vi "connect.vi"(0 "username":string="user", 5 "password":string="password", 7 "host":string="localhost", 9 "port":i32=33060, 11 "error in (no error)":errorcluster) -> (4 "DB Session ID":i32, 15 "error out":errorcluster)   [LabVIEW 2017, in "Database.lvlib"]
uses:
  Database.lvlib
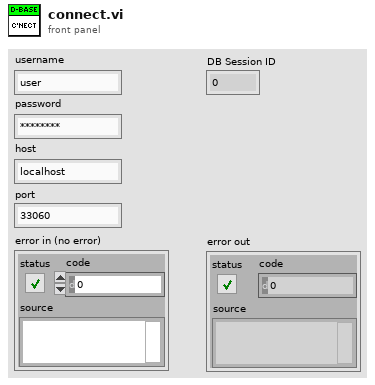
[diagram p1: front panel]
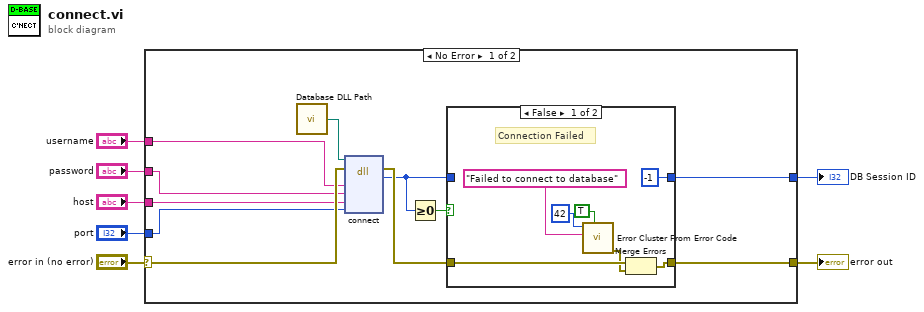
[diagram p0: block diagram]
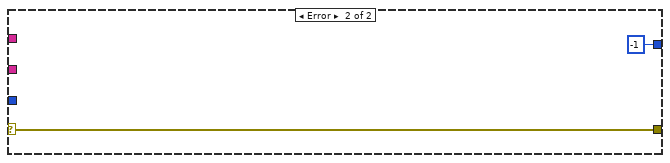
[diagram p3: hidden frame]
diagram:
  n1 = case shown="No Error" "error in (no error)" {
    selector: "error in (no error)" -> [w18 w29]
    tunnel: [w14 w29] -> w6
    tunnel: "username" -> [w11 _]
    tunnel: "password" -> [w10 _]
    tunnel: "host" -> [w9 _]
    tunnel: "port" -> [w8 _]
    tunnel: [w13 -1 ("return type")] -> w1
    frame No Error {
      n2 = call "Database DLL Path.vi"() -> ("DLL Path"=w12:path)  [unwired: 5 in]
      n3 = dll-call lib="?" fn="connect"(path in=w12, error in=w18, "username"=w11, "password"=w10, "url"=w9, "port"=w8) -> (error out=w16:errorcluster, "return type"=w15:i32)  [unwired: 5 in, 1 out]
      n4 = Greater Or Equal To 0?(x=w15) -> (x >= 0?=w17:bool)
      n5 = case shown="False" w17 {
        tunnel: w16 -> [w24 w26]
        tunnel: w15 -> [_ w27]
        tunnel: [-1 ("return type") w27] -> w13
        tunnel: [w23 w26] -> w14
        frame False {
          # "Connection Failed"
          n6 = call <vilib>:"Error Cluster From Error Code.vi"("show call chain? (False)"=TRUE, "error message (\"\")"="Failed to connect to database" ("error message (\"\")"), "error code (0)"=42) -> ("error out"=w22:errorcluster)  [unwired: 6 in]
          n7 = Merge Errors(w24, w22) -> (w23:errorcluster)
        }
        frame True {
          # "Connection Successful"
        }
      }
    }
    frame Error {
    }
  }
  "error out" <- w6
  "DB Session ID" <- w1
